vi "Spectrometer Digikröm.vi"(8 "error in (no error)":errorcluster, 11 "Spectrometer Digikröm in":refnum<class "Spectrometer Digikröm.lvclass">) -> (0 "error out":errorcluster, 3 "Spectrometer Digikröm out":refnum<class "Spectrometer Digikröm.lvclass">)   [LabVIEW 2017, in "Spectrometer Digikröm.lvclass"]
uses:
  Global/GPIB Numbers.vi
panel:
  out "Status":string
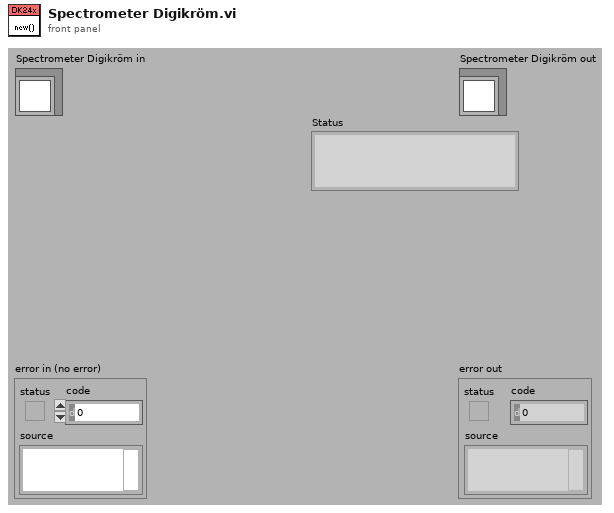
[diagram p1: front panel]
types:
  T1 = typedef "GPIB Type Def.ctl" = cluster{"Name":string, "bus":dbl, "GPIB":dbl, "GPIB as string":string, "byte":i32, "VISA Resource Name":refnum<visa-resource-name>}
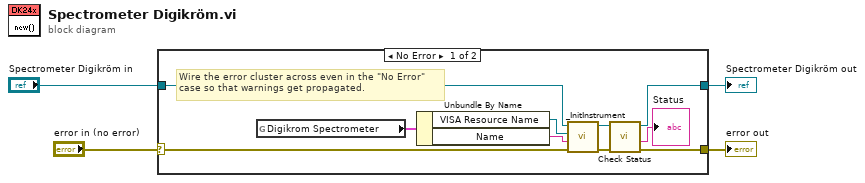
[diagram p0: block diagram]
diagram:
  n1 = case shown="No Error" "error in (no error)" {
    selector: "error in (no error)" -> [w10 w16]
    tunnel: [w6 w16] -> w3
    tunnel: [w8 w15] -> w1
    tunnel: "Spectrometer Digikröm in" -> [w14 w15]
    frame No Error {
      # "Wire the error cluster across even in the \"No Error\"\ncase so that warnings get propagated."
      n2 = global read "GPIB Numbers.vi" "Digikrom Spectrometer"() -> (w13:T1)
      n3 = Unbundle By Name(w13) -> ("VISA Resource Name"=w12:refnum<visa-resource-name>, "Name"=w11:string)
      n4 = call-dynamic "_InitInstrument.vi"("error in (no error)"=w10, "Name"=w11, "VISA Resource Name"=w12, "Instrument in"=w14) -> ("error out"=w7:errorcluster, "Instrument out"=w9:refnum<class "Spectrometer Digikröm.lvclass">)  [unwired: 2 in, 4 out]
      n5 = call-dynamic "Check Status.vi"("error in (no error)"=w7, "Spectrometer Digikröm in"=w9) -> ("error out"=w6:errorcluster, "Status"=→"Status":string, "Spectrometer Digikröm out"=w8:refnum<class "Spectrometer Digikröm.lvclass">)  [unwired: 6 in, 1 out]
    }
    frame Error {
    }
  }
  "error out" <- w3
  "Spectrometer Digikröm out" <- w1
